vi "Set Test Step .vi"(8 "error in (no error)":errorcluster, 10 "Current Step":T1, 11 "Sequence Context In":refnum<k7>) -> (0 "error out":errorcluster, 1 "Next Step":i32, 2 "Test Running":bool, 3 "HV":bool)   [LabVIEW 2021, in "TestExec.lvclass"]
uses:
  TestExec.lvclass
  Controls/Rx TestExec.ctl
  <vilib>/addons/TestStand/_TSUtility.llb/TestStand - Set Property Value (Number {Unsigned 32-bit Integer}).vi
  <vilib>/addons/TestStand/_TSUtility.llb/TestStand - Get Property Value (Number {Signed 32-bit Integer}).vi
  TestExec.lvclass/TestExec.ctl
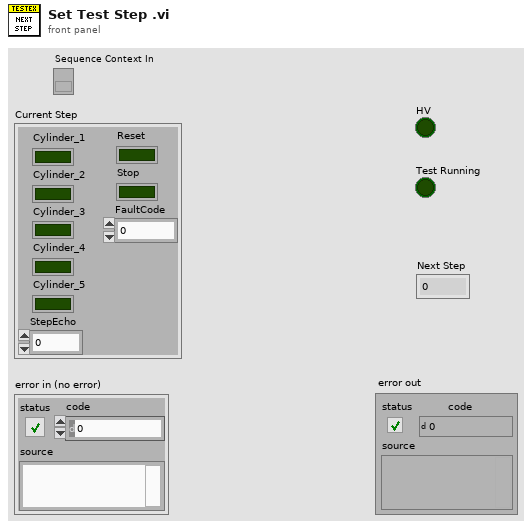
[diagram p1: front panel]
types:
  T1 = typedef "TestExec.lvclass/Rx TestExec.ctl" = cluster{"Cylinder_1":bool, "Cylinder_2":bool, "Cylinder_3":bool, "Cylinder_4":bool, "Cylinder_5":bool, "StepEcho":u32, "Reset":bool, "Stop":bool, "FaultCode":u32}
  T2 = typedef "TestStand - Status Monitor.ctl" = cluster{"Sequence Context":refnum<k7>, "Execution":refnum<k7>, "Termination Monitor":refnum<k7>}
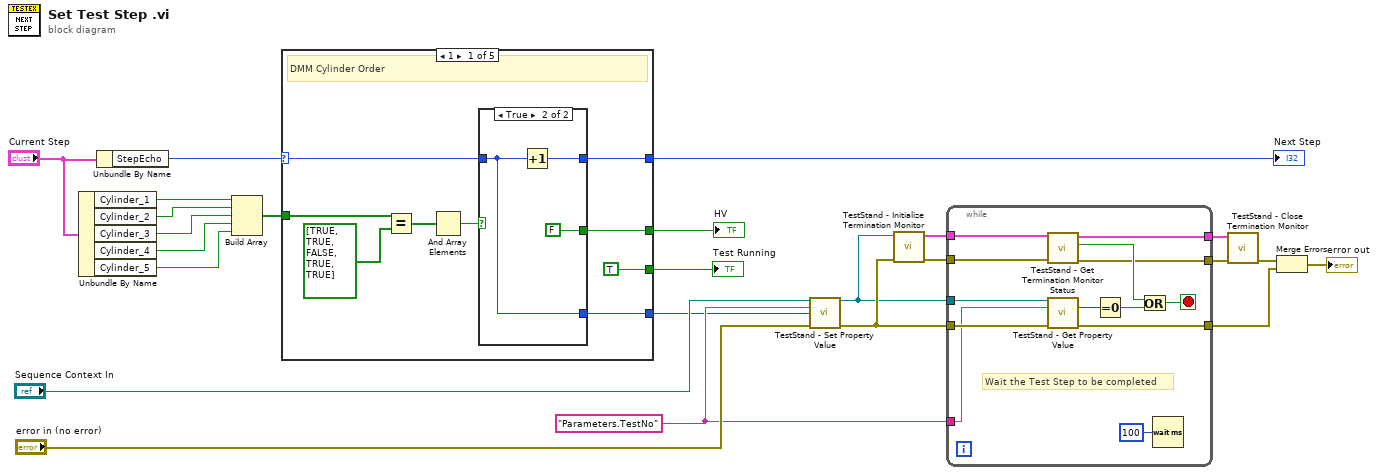
[diagram p0: block diagram]
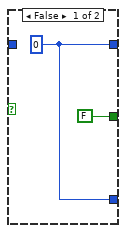
[diagram p2: hidden frame]
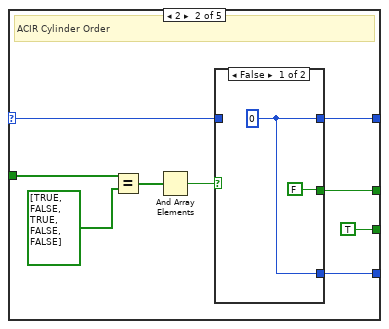
[diagram p3: hidden frame]
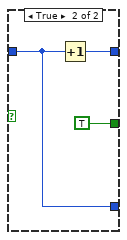
[diagram p4: hidden frame]
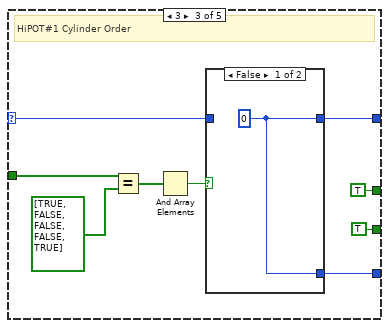
[diagram p5: hidden frame]
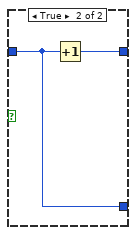
[diagram p6: hidden frame]
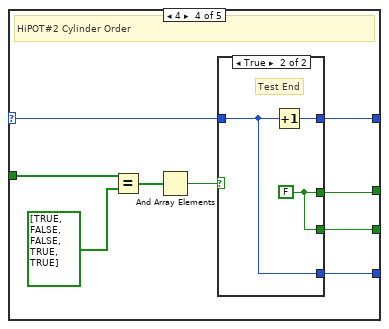
[diagram p7: hidden frame]
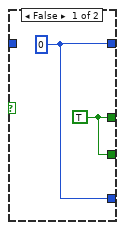
[diagram p8: hidden frame]
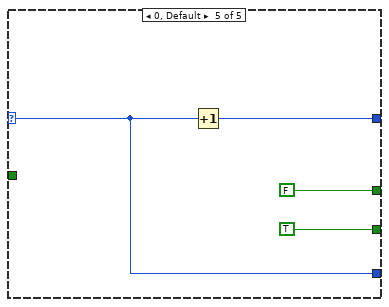
[diagram p9: hidden frame]
diagram:
  w10 = "Parameters.TestNo" ("Lookup String")
  n1 = Unbundle By Name("Current Step") -> ("Cylinder_1"=w23:bool, "Cylinder_2"=w22:bool, "Cylinder_3"=w21:bool, "Cylinder_4"=w20:bool, "Cylinder_5"=w19:bool)
  n2 = Unbundle By Name("Current Step") -> ("StepEcho"=w18:u32)
  n3 = Build Array(w23, w22, w21, w20, w19) -> (w17:bool[])
  n4 = case shown="1" w18 {
    selector: w18 -> [w31 w44 w57 w66 w79]
    tunnel: w17 -> [w26 w40 w54 w72 _]
    tunnel: [w28 w43 w56 w65 w80] -> w16
    tunnel: [w29 w42 TRUE w69 FALSE] -> w15
    tunnel: [TRUE ("Test Running") TRUE ("Test Running") TRUE ("Test Running") w68 TRUE ("Test Running")] -> w14
    tunnel: [w25 w39 w55 w67 w79] -> w9
    frame 1 {
      # "DMM Cylinder Order"
      n5 = Equal?(x=w26, y=bool[] [TRUE, TRUE, FALSE, TRUE, TRUE]) -> (x = y?=w33:bool[])
      n6 = And Array Elements(Boolean array=w33) -> (logical AND=w30:bool)
      n7 = case shown="True" w30 {
        tunnel: w31 -> [_ w36]
        tunnel: [w34 w38] -> w28
        tunnel: [FALSE FALSE] -> w29
        tunnel: [w34 w36] -> w25
        frame False {
          w34 = 0
        }
        frame True {
          n8 = Increment(x=w36) -> (x+1=w38:u32)
        }
      }
    }
    frame 2 {
      # "ACIR Cylinder Order"
      n9 = Equal?(x=w40, y=bool[] [TRUE, FALSE, TRUE, FALSE, FALSE]) -> (x = y?=w47:bool[])
      n10 = And Array Elements(Boolean array=w47) -> (logical AND=w45:bool)
      n11 = case shown="False" w45 {
        tunnel: w44 -> [_ w50]
        tunnel: [w48 w52] -> w43
        tunnel: [FALSE TRUE] -> w42
        tunnel: [w48 w50] -> w39
        frame False {
          w48 = 0
        }
        frame True {
          n12 = Increment(x=w50) -> (x+1=w52:u32)
        }
      }
    }
    frame 3 {
      # "HiPOT#1 Cylinder Order"
      n13 = Equal?(x=w54, y=bool[] [TRUE, FALSE, FALSE, FALSE, TRUE]) -> (x = y?=w61:bool[])
      n14 = And Array Elements(Boolean array=w61) -> (logical AND=w58:bool)
      n15 = case shown="False" w58 {
        tunnel: w57 -> [_ w63]
        tunnel: [w62 w64] -> w56
        tunnel: [w62 w63] -> w55
        frame False {
          w62 = 0
        }
        frame True {
          n16 = Increment(x=w63) -> (x+1=w64:u32)
        }
      }
    }
    frame 4 {
      # "HiPOT#2 Cylinder Order"
      n17 = Equal?(x=w72, y=bool[] [TRUE, FALSE, FALSE, TRUE, TRUE]) -> (x = y?=w73:bool[])
      n18 = And Array Elements(Boolean array=w73) -> (logical AND=w70:bool)
      n19 = case shown="True" w70 {
        tunnel: [w75 w78] -> w69
        tunnel: [w75 w78] -> w68
        tunnel: [w74 w77] -> w67
        tunnel: w66 -> [_ w77]
        tunnel: [w74 w76] -> w65
        frame False {
          w74 = 0 ("StepEcho")
          w75 = TRUE
        }
        frame True {
          w78 = FALSE
          # "Test End"
          n20 = Increment(x=w77) -> (x+1=w76:u32)
        }
      }
    }
    frame 0, Default {
      n21 = Increment(x=w79) -> (x+1=w80:u32)
    }
  }
  "Next Step" <- w16
  "HV" <- w15
  "Test Running" <- w14
  n22 = call-poly <vilib>:"TestStand - Set Property Value.vi"("Sequence Context In"="Sequence Context In", "Lookup String"=w10, "New Value"=w9, "error in (no error)"="error in (no error)") -> ("Sequence Context Out"=w8:refnum<k7>, "error out"=w11:errorcluster)  [unwired: 10 in]
  n23 = call <vilib>:"TestStand - Initialize Termination Monitor.vi"("error in (no error)"=w11, "Sequence Context In"=w8) -> ("error out"=w3:errorcluster, "Status Monitor Out"=w4:T2)  [unwired: 8 in]
  n24 = while {
    tunnel: w8 -> [w95]
    tunnel: w11 -> [w94]
    tunnel: w10 -> [w92]
    tunnel: [w90] -> w6
    tunnel: w4 -> [w89]
    tunnel: [w88] -> w1
    tunnel: w3 -> [w87]
    tunnel: [w83] -> w2
    stop <- w84 stop-if-true
    # "Wait the Test Step to be completed"
    n25 = call <vilib>:"TestStand - Get Termination Monitor Status.vi"("error in (no error)"=w87, "Status Monitor In"=w89) -> ("error out"=w83:errorcluster, "Terminating or Aborting"=w86:bool, "Status Monitor Out"=w88:T2)  [unwired: 7 in]
    n26 = call-poly <vilib>:"TestStand - Get Property Value.vi"("Sequence Context In"=w95, "Lookup String"=w92, "error in (no error)"=w94) -> ("Value"=w93:i32, "error out"=w90:errorcluster)  [unwired: 10 in, 1 out]
    n27 = Equal To 0?(x=w93) -> (x = 0?=w85:bool)
    n28 = Or(x=w86, y=w85) -> (x .or. y?=w84:bool)
    n29 = Wait (ms)(milliseconds to wait=u32 100) -> ()  [unwired: 1 out]
  }
  n30 = call <vilib>:"TestStand - Close Termination Monitor.vi"("error in (no error)"=w2, "Status Monitor In"=w1) -> ("error out"=w7:errorcluster)  [unwired: 9 in]
  n31 = Merge Errors(w7, w6) -> (→"error out":errorcluster)
